vi "Adv_GetData.vi"(8 "error in (no error)":errorcluster, 10 "IImageDataSet":refnum<k24>, 11 "LightField Automation in":refnum<class "LightField Automation.lvclass">) -> (0 "error out":errorcluster, 2 "Data":T1(array[cluster]), 3 "LightField Automation out":refnum<class "LightField Automation.lvclass">)   [LabVIEW 2013, in "LightField Automation.lvclass"]
uses:
  LightField Automation.lvclass
  C:/Program Files/Princeton Instruments/LightField/AddInViews/PrincetonInstruments.LightFieldViewV3.dll
  Program Files/Princeton Instruments/LightField/AddInViews/PrincetonInstruments.LightFieldViewV3.dll
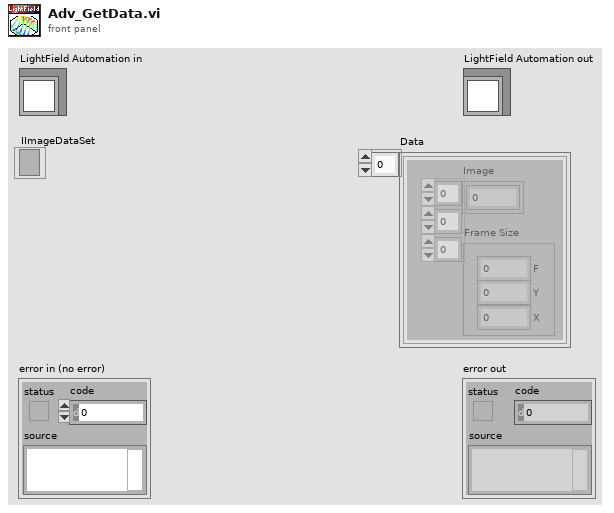
[diagram p1: front panel]
types:
  T1 = cluster{"Image":dbl[][][], "Frame Size":cluster{"F":i32, "Y":i32, "X":i32}}[]
  T2 = cluster{"Image":dbl[][][], "Frame Size":cluster{"F":i32, "Y":i32, "X":i32}}
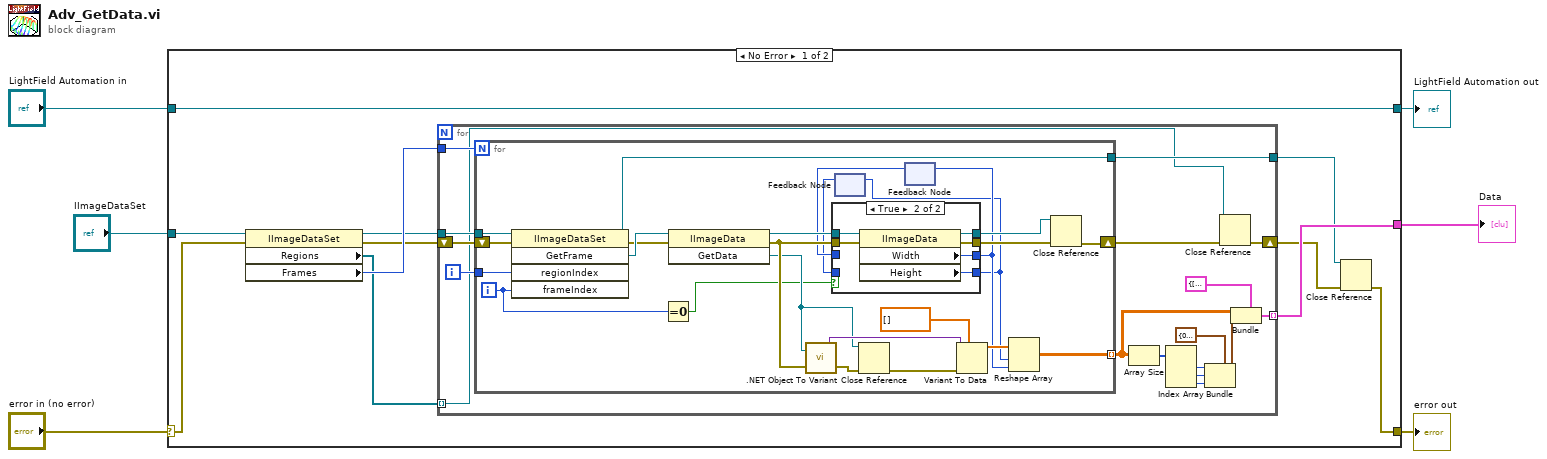
[diagram p0: block diagram]
diagram:
  n1 = case shown="No Error" "error in (no error)" {
    selector: "error in (no error)" -> [w8 w70]
    tunnel: [w15 w70] -> w5
    tunnel: [w7 w69] -> w3
    tunnel: "LightField Automation in" -> [w7 w69]
    tunnel: [w17 _] -> w2
    tunnel: "IImageDataSet" -> [w9 _]
    frame No Error {
      n2 = property class="IImageDataSet"(reference=w9, error in=w8) -> (reference out=w11:refnum<k24>, error out=w12:errorcluster, "Regions"=w10:refnum<k24>[], "Frames"=w13:i64)
      n3 = for {
        tunnel: w11 -> [w34]
        shift-right: [w19] -> w16
        shift-left: w12 -> [w33]
        tunnel: w13 -> [w32]
        tunnel: [w28] -> w17 mode=indexing
        tunnel: [w21] -> w14
        tunnel: w10 -> [w18] mode=indexing
        i -> [w31]
        n4 = for {
          N: w32 -> [_]
          tunnel: w34 -> [w48]
          tunnel: w31 -> [w57]
          shift-right: [w45] -> w20
          shift-left: w33 -> [w58]
          tunnel: [w49] -> w29 mode=indexing
          tunnel: [w44] -> w21
          i -> [w40]
          n5 = invoke class="IImageDataSet" method="GetFrame"(reference=w48, error in=w58, "regionIndex"=w57, "frameIndex"=w40) -> (reference out=w44:refnum<k24>, error out=w55:errorcluster, "GetFrame"=w56:refnum<k24>)  [unwired: 1 in, 2 out]
          n6 = Equal To 0?(x=w40) -> (x = 0?=w39:bool)
          n7 = invoke class="IImageData" method="GetData"(reference=w56, error in=w55) -> (reference out=w54:refnum<k24>, error out=w53:errorcluster, "GetData"=w41:refnum<k24>)  [unwired: 1 in]
          n8 = call <vilib>:".NET Object To Variant.vi"("error in (no error)"=w53, ".NET object"=w41) -> ("error out"=w42:errorcluster, "variant"=w52:variant)
          n9 = feedback #1() -> (w35:i32)  [unwired: 1 in]
          n10 = Close Reference(reference=w41, error in (no error)=w42) -> (error out=w43:errorcluster)
          n11 = feedback #2() -> (w36:i32)  [unwired: 1 in]
          n12 = case shown="True" w39 {
            tunnel: w54 -> [w62 w68]
            tunnel: w53 -> [w61 w67]
            tunnel: [w60 w66] -> w38
            tunnel: [w59 w65] -> w37
            tunnel: [w61 w64] -> w47
            tunnel: [w62 w63] -> w46
            tunnel: w36 -> [w60 _]
            tunnel: w35 -> [w59 _]
            frame False {
            }
            frame True {
              n13 = property class="IImageData"(reference=w68, error in=w67) -> (reference out=w63:refnum<k24>, error out=w64:errorcluster, "Width"=w66:i32, "Height"=w65:i32)
            }
          }
          n14 = feedback-in #1(w37) -> ()
          n15 = feedback-in #2(w38) -> ()
          n16 = Variant To Data(error in=w43, type=dbl[] [], Variant=w52) -> (data=w50:dbl[])  [unwired: 1 out]
          n17 = Reshape Array(w50, w37, w38) -> (w49:dbl[][])
          n18 = Close Reference(reference=w46, error in (no error)=w47) -> (error out=w45:errorcluster)
        }
        n19 = Array Size(array=w29) -> (size(s)=w30:i32[])
        n20 = Index Array(array=w30) -> (element #1=w26:i32, element #2=w27:i32, element #3=w25:i32)  [unwired: 3 in]
        n21 = Bundle(cluster=cluster{"F":i32, "Y":i32, "X":i32} {"F"=0, "Y"=0, "X"=0} ("Frame Size"), "F"=w26, "Y"=w27, "X"=w25) -> (w22:cluster{"F":i32, "Y":i32, "X":i32})
        n22 = Close Reference(reference=w18, error in (no error)=w20) -> (error out=w19:errorcluster)
        n23 = Bundle(cluster=T2 {"Image"=[], "Frame Size"={"F"=0, "Y"=0, "X"=0}} ("Cluster"), "Image"=w29, "Frame Size"=w22) -> (w28:T2)
      }
      n24 = Close Reference(reference=w14, error in (no error)=w16) -> (error out=w15:errorcluster)
    }
    frame Error {
    }
  }
  "error out" <- w5
  "LightField Automation out" <- w3
  "Data" <- w2
